vi "Call_LibSO.vi"() -> ()   [LabVIEW 2014]
uses:
  libhello.so
panel:
  out "return type":i32
  out "Sub":i32
  in  "b":i32
  in  "a":i32
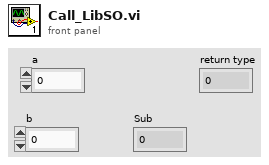
[diagram p1: front panel]
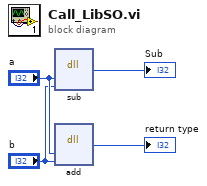
[diagram p0: block diagram]
diagram:
  n1 = dll-call lib="libhello.so" fn="sub"("a"="a", "b"="b") -> ("return type"=→"Sub":i32)  [unwired: 5 in, 2 out]
  n2 = dll-call lib="libhello.so" fn="add"("a"="a", "b"="b") -> ("return type"=→"return type":i32)  [unwired: 5 in, 2 out]
